vi "Reset.vi"(8 "error in (no error)":errorcluster, 11 "SQL Statement in":refnum<class "SQL Statement.lvclass">) -> (0 "error out":errorcluster, 3 "SQL Statement out":refnum<class "SQL Statement.lvclass">)   [LabVIEW 2011, in "SQLite.lvlib" / "SQL Statement.lvclass"]
doc: "Resets an prepared SQL statement to its initial state before execution. Note that this does not clear any bound parameters.\n\nThis VI will operate even if an error is input into the \"error in\" terminal. Unlike with the C interface \"sqlite3_reset\" command, this VI does NOT return the error code of the previously executed \"step\"."
uses:
  SQL Statement.lvclass
  SQL Statement.lvclass/SQL Statement.ctl
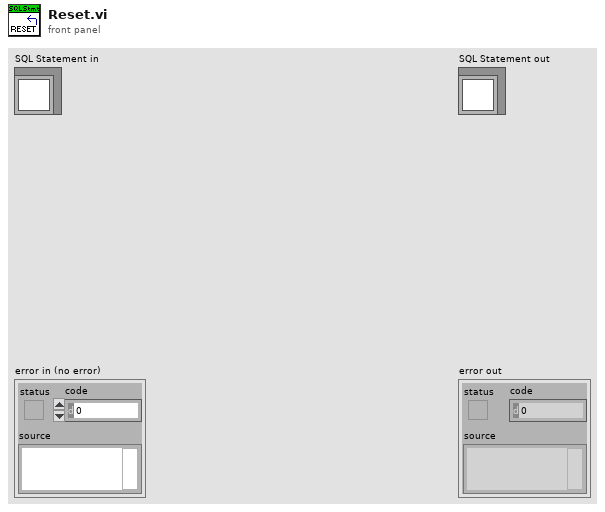
[diagram p1: front panel]
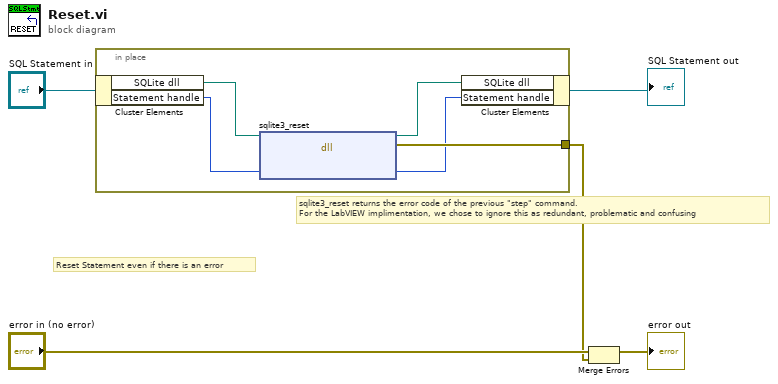
[diagram p0: block diagram]
diagram:
  # "sqlite3_reset returns the error code of the previous \"step\" command.\nFor the LabVIEW implimentation, we chose to ignore this as redundant, problematic and confusing"
  # "Reset Statement even if there is an error"
  n1 = in-place {
    in-place-border: [w10] -> w3
    n2 = in-place-cluster #1("SQL Statement in") -> ("SQLite dll"=w9:path, "Statement handle"=w8:u64)
    n3 = dll-call lib="C:/SQLite/sqlite3.dll" fn="sqlite3_reset"(path in=w9, "Statement"=w8) -> (path out=w6:path, error out=w10:errorcluster, "Statement"=w7:u64)  [unwired: 3 in]
    n4 = in-place-cluster #1("SQLite dll"=w6, "Statement handle"=w7) -> (→"SQL Statement out":refnum<class "SQL Statement.lvclass">)
  }
  n5 = Merge Errors("error in (no error)", w3) -> (→"error out":errorcluster)
